vi "SaveFrontPanelCapture.vi"(4 "Option":T1={"JPG Quqlity(80)"=80, "PNG Comp(-1)"=-1}, 5 "Cut Border":T2={"Left"=1, "Up"=1, "Right"=1, "Down"=1}, 6 "Format":enum16{"JPG", "PNG", "BMP"}(ring), 7 "Image Path":path, 8 "error in (no error)":errorcluster caption="エラー入力（エラーなし）", 10 "Bit Depth":i32, 11 "リファレンス":refnum<vi>) -> (0 "error out":errorcluster caption="エラー出力")   [LabVIEW 2014]
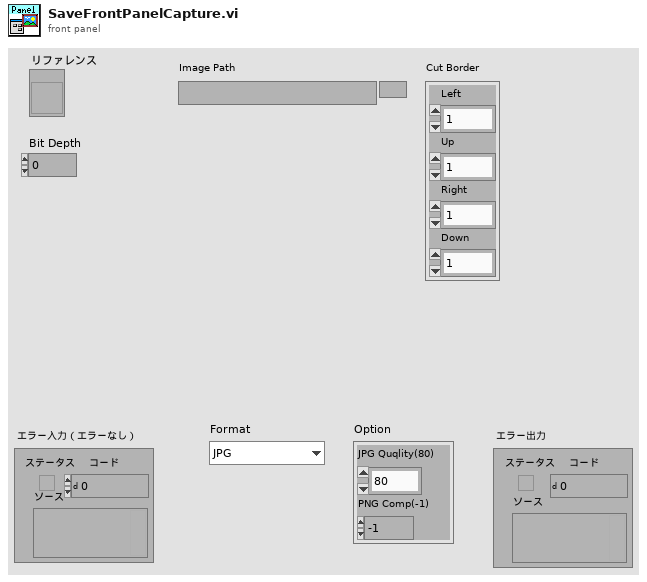
[diagram p1: front panel]
types:
  T1 = cluster{"JPG Quqlity(80)":i32, "PNG Comp(-1)":i32}
  T2 = cluster{"Left":i16, "Up":i16, "Right":i16, "Down":i16}
  T3 = typedef "imagedata.ctl" = cluster{"image type":i32, "image depth":i32, "image":u8[], "mask":u8[], "colors":u32[], "Rectangle":cluster{"left":i16, "top":i16, "right":i16, "bottom":i16}}
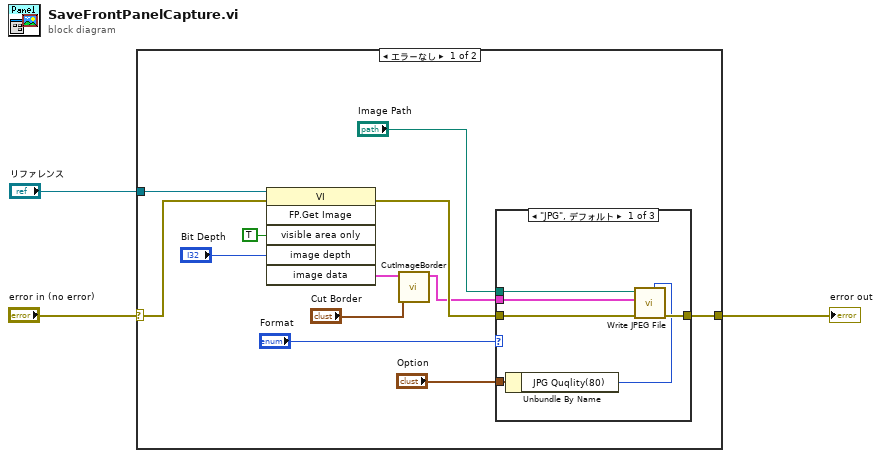
[diagram p0: block diagram]
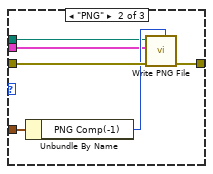
[diagram p2: hidden frame]
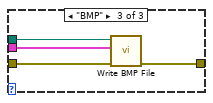
[diagram p3: hidden frame]
diagram:
  n1 = case shown="エラーなし" "error in (no error)" {
    selector: "error in (no error)" -> [w12 w32]
    tunnel: [w6 w32] -> w2
    tunnel: "リファレンス" -> [w13 _]
    frame No Error {
      n2 = invoke class="VI" method="FP.Get Image"(reference=w13, error in=w12, "visible area only"=TRUE ("可視領域のみ"), "image depth"="Bit Depth") -> (error out=w5:errorcluster, "image data"=w10:T3)  [unwired: 2 in, 4 out]
      n3 = call "CutImageBorder.vi"("削除枠幅"="Cut Border", "元画像"=w10) -> ("切抜き画像"=w4:T3)  [unwired: 9 in]
      n4 = case shown="\"JPG\", デフォルト" "Format" {
        tunnel: [w21 w27 w28] -> w6
        tunnel: w5 -> [w20 w26 w31]
        tunnel: "Image Path" -> [w19 w23 w30]
        tunnel: w4 -> [w18 w22 w29]
        tunnel: "Option" -> [w17 w25 _]
        frame "JPG", Default {
          n5 = Unbundle By Name(w17) -> ("JPG Quqlity(80)"=w16:i32)
          n6 = call <vilib>:"Write JPEG File.vi"("quality (80)"=w16, "error in (no error)"=w20, "image data"=w18, "path to JPEG file"=w19) -> ("error out"=w21:errorcluster)  [unwired: 6 in, 1 out]
        }
        frame "PNG" {
          n7 = Unbundle By Name(w25) -> ("PNG Comp(-1)"=w24:i32)
          n8 = call <vilib>:"Write PNG File.vi"("compression (default)"=w24, "error in (no error)"=w26, "image data"=w22, "path to PNG file"=w23) -> ("error out"=w27:errorcluster)  [unwired: 6 in, 1 out]
        }
        frame "BMP" {
          n9 = call <vilib>:"Write BMP File.vi"("error in (no error)"=w31, "image data"=w29, "path to BMP file"=w30) -> ("error out"=w28:errorcluster)  [unwired: 7 in, 1 out]
        }
      }
    }
    frame Error {
    }
  }
  "error out" <- w2
